vi "TEST1.vi"() -> ()   [LabVIEW 2014]
panel:
  in  "stop 2":bool
  in  "stop":bool
  out "Indicator":bool
  in  "Indicator":bool
  # "BOMET COMMUNICATION TEST"
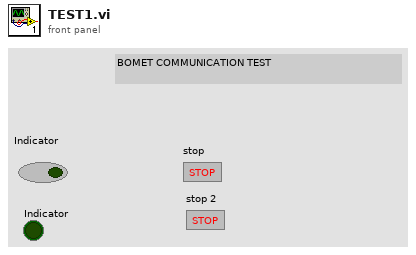
[diagram p1: front panel]
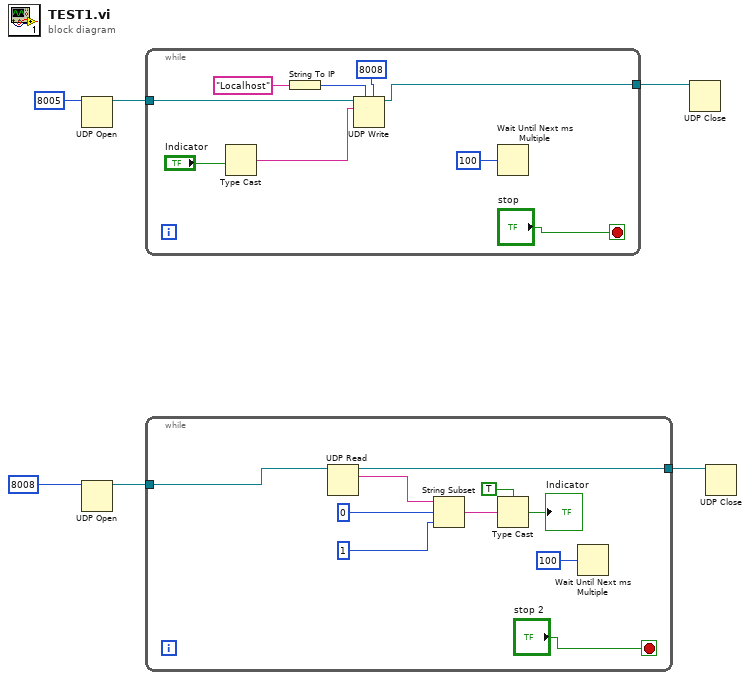
[diagram p0: block diagram]
diagram:
  n1 = UDP Open(11:u16 8005 ("port")) -> (port=w5:refnum<k16>)  [unwired: 4 in, 2 out]
  n2 = UDP Open(11:u16 8008 ("port")) -> (port=w3:refnum<k16>)  [unwired: 4 in, 2 out]
  n3 = while {
    tunnel: w5 -> [w15]
    tunnel: [w14] -> w4
    stop <- "stop" stop-if-true
    n4 = Type Cast(x="Indicator") -> (*(type *) &x=w9:string)  [unwired: 1 in]
    n5 = String To IP(1:"Localhost" ("name")) -> (0:w12:u32)
    n6 = UDP Write(address=w12, port or service name=u16 8008, connection ID=w15, data in=w9) -> (3:w14:refnum<k16>)  [unwired: 2 in, 1 out]
    n7 = Wait Until Next ms Multiple(millisecond multiple=u32 100) -> ()  [unwired: 1 out]
  }
  n8 = while {
    tunnel: w3 -> [w25]
    tunnel: [w24] -> w2
    stop <- "stop 2" stop-if-true
    n9 = UDP Read(connection ID=w25) -> (data out=w23:string, 3:w24:refnum<k16>)  [unwired: 3 in, 3 out]
    n10 = String Subset(string=w23, offset (0)=0, length (rest)=1 ("offset (0)")) -> (substring=w19:string)
    n11 = Type Cast(type=TRUE, x=w19) -> (*(type *) &x=→"Indicator":bool)
    n12 = Wait Until Next ms Multiple(millisecond multiple=u32 100) -> ()  [unwired: 1 out]
  }
  n13 = UDP Close(connection ID=w4) -> ()  [unwired: 1 in, 2 out]
  n14 = UDP Close(connection ID=w2) -> ()  [unwired: 1 in, 2 out]
